vi "SetRequestContinousAquisition.vi"(0 "object in":refnum<class "Hamamatsu.lvclass">, 1 "RequestContinousAquisition?":bool, 5 "error in (no error)":errorcluster) -> (14 "object out":refnum<class "Hamamatsu.lvclass">, 19 "error out":errorcluster)   [LabVIEW 2021, in "Hamamatsu.lvclass"]
uses:
  Hamamatsu.lvclass
  Hamamatsu.lvclass/Hamamatsu.ctl
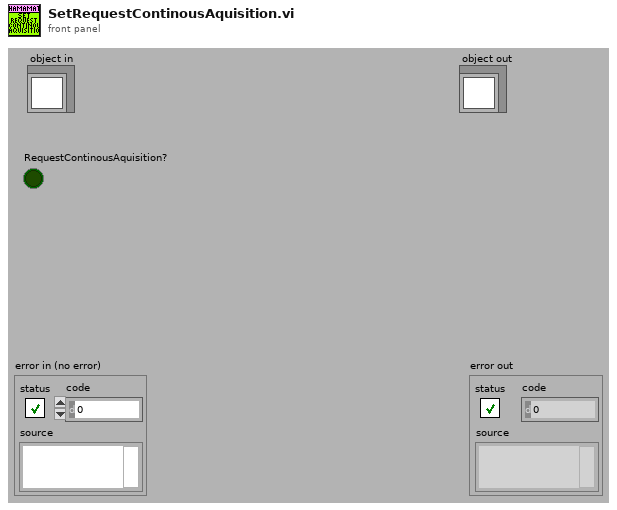
[diagram p1: front panel]
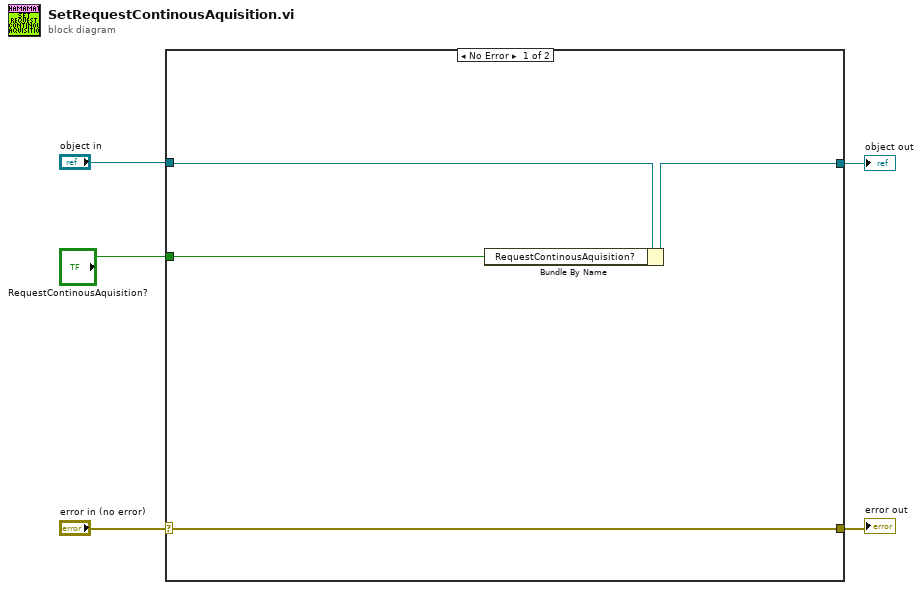
[diagram p0: block diagram]
diagram:
  n1 = case shown="No Error" "error in (no error)" {
    selector: "error in (no error)" -> [w8 w11]
    tunnel: [w8 w11] -> w4
    tunnel: [w6 w10] -> w2
    tunnel: "object in" -> [w7 w10]
    tunnel: "RequestContinousAquisition?" -> [w9 _]
    frame No Error {
      n2 = Bundle By Name(cluster=w7, "RequestContinousAquisition?"=w9) -> (w6:refnum<class "Hamamatsu.lvclass">)
    }
    frame Error {
    }
  }
  "error out" <- w4
  "object out" <- w2
